vi "MeasureDistanceGantryCalibCheck.vi"() -> ()   [LabVIEW 2019]
uses:
  <vilib>/userDefined/High Color/IMAQdx.ctl
  include/GlobalVariables.vi
  Other Models/2010/Motion/AbortSingle.vi
  <vilib>/vision/driver/NI_Vision_Acquisition_Software.lvlib
panel:
  in  "TemplateFileName":string="C:\\Users\\TTUHEP\\Pictures\\SiCorner.png"
  out "X2Y2":string
  out "X1Y1":string
  in  "ObjectDetType":enum16{"Pattern", "ManualPick", "FidCircle"}(ring)
  in  "Gcode2":string="G90\nG1 Z0 F100\nG1 X224.526 Y907.397 F100//Si corner on BP A1\nG1 Z68.674 F100//Si Corner on BP A1\n//G1 X194.1280 Y755.823 F100 //Si Corner on BP A2\r//G1 Z68.8520934 //Si Corner on BP A1"
  in  "EnablePoint1":bool
  in  "Gcode1":string="G90\nG1 Z0 F100\nG1 X850.587 Y914.513 F100//Si corner A1\nG1 Z75.21 F100//Si Corner A1\n//G1 X768.633 Y750.333 F100 //Si corner A2\r//G1 Z75.0621//Si corner A2"
  in  "Operation2":enum16{"JoyStick", "FixedXY"}(ring)
  in  "Operation1":enum16{"JoyStick", "FixedXY"}(ring)
  out "CamX1Y1X2Y2Dist":string
  out "DistanceCam":dbl
  out "CamY 2":dbl
  out "CamX 2":dbl
  out "CamY":dbl
  out "CamX":dbl
  in  "EnablePoint2":bool
  out "error out":errorcluster
  out "X1Y1X2Y2Dist":string
  out "Distance":dbl
  out "Y2":dbl format="%#_7g"
  out "X2":dbl
  out "Radius 2":dbl
  out "CenterPosition 2":cluster{"X":sgl, "Y":sgl}
  in  "StopJoyStick 2":bool
  out "Image 2":T1(plugin-control)
  out "Y1":dbl format="%#_7g"
  out "X1":dbl
  out "Radius":dbl
  out "CenterPosition":cluster{"X":sgl, "Y":sgl}
  in  "StopJoyStick":bool
  in  "Autofocus":T2={"Enable"=TRUE, "InitialStepSize"=0.05, "Tolerance"=0.02, "Abort"=FALSE} {"Tolerance" format="%#_13g"}
  out "Image":T1(plugin-control)
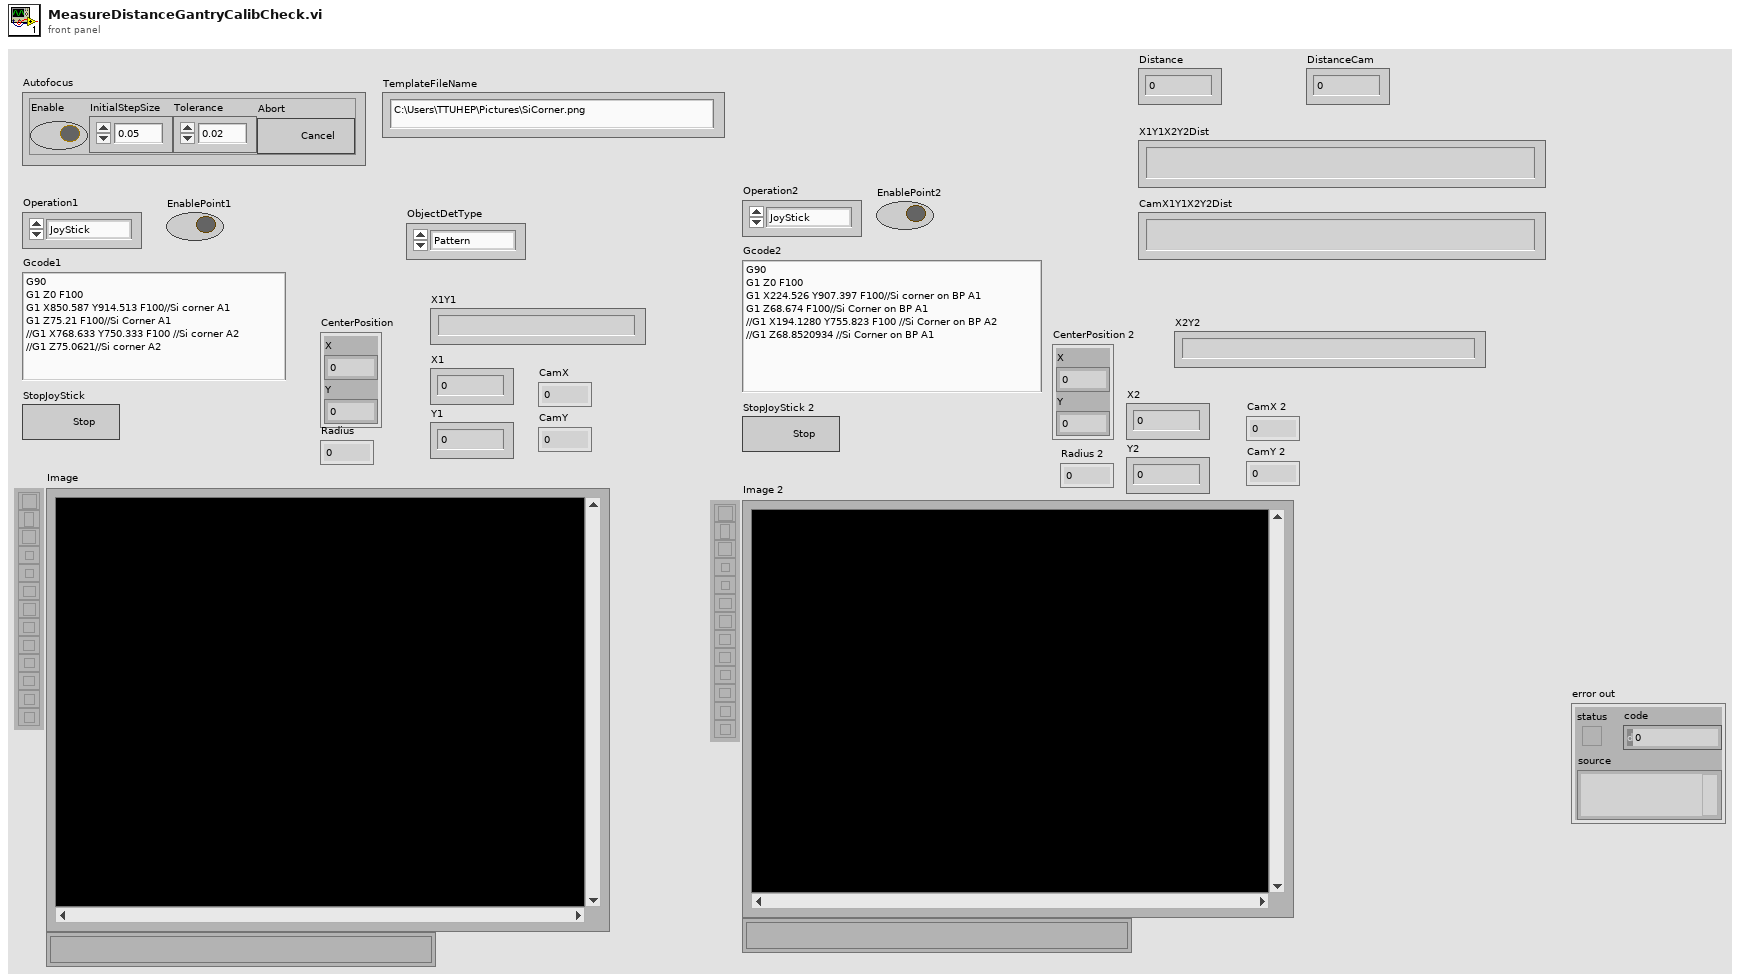
[diagram p1: front panel]
types:
  T1 = typedef "IMAQ Image.ctl" = refnum<image>
  T2 = cluster{"Enable":bool, "InitialStepSize":dbl, "Tolerance":dbl, "Abort":bool}
  T3 = typedef "IMAQdx.ctl" = refnum<k21>
  T4 = typedef "Image Type" = u32
  T5 = typedef "IMAQ Point" = cluster{"X":sgl, "Y":sgl}
  T6 = cluster{"Position":cluster{"X":sgl, "Y":sgl}, "Radius":dbl, "Score":dbl}
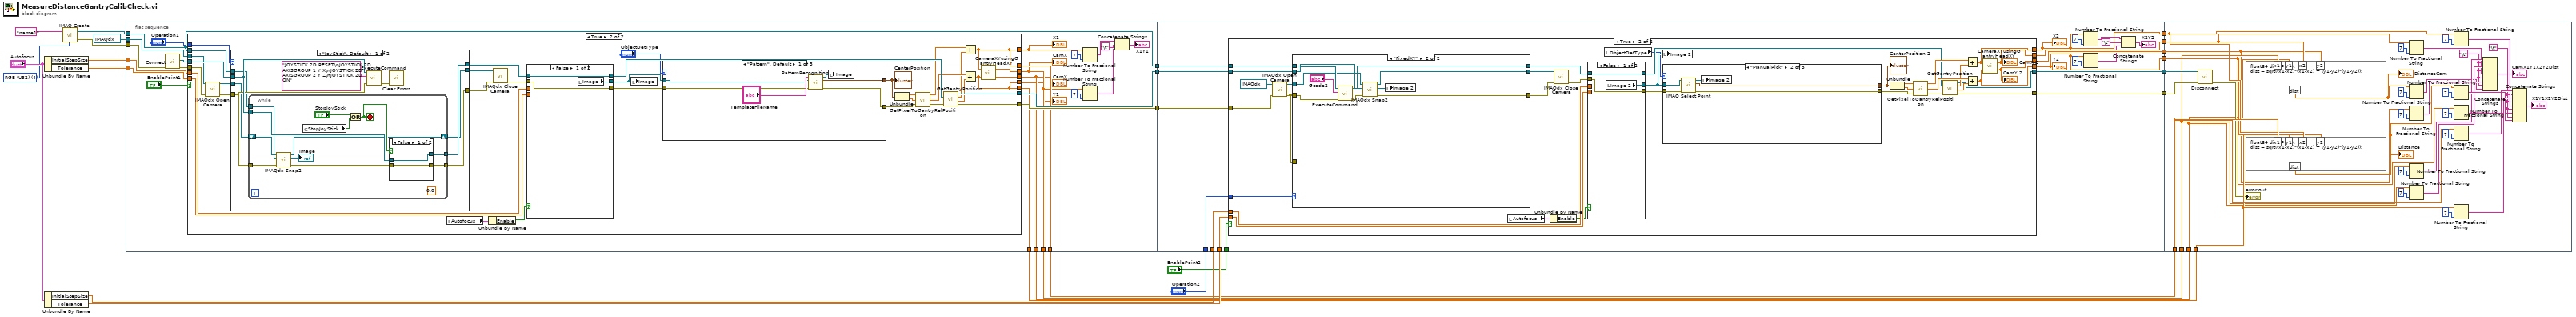
[diagram p0: block diagram]
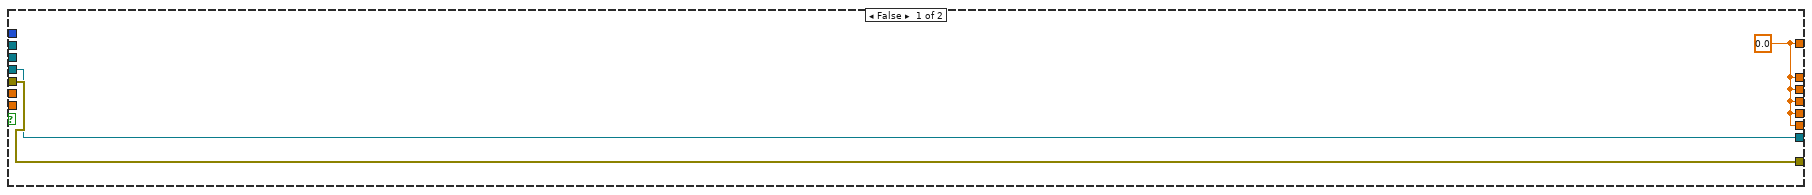
[diagram p2: hidden frame]
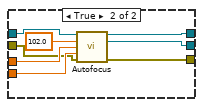
[diagram p3: hidden frame]
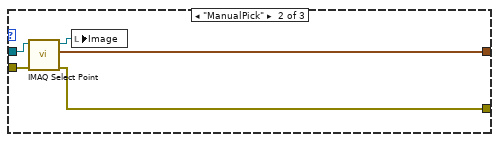
[diagram p4: hidden frame]
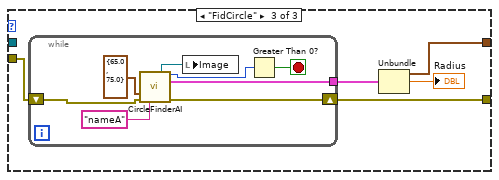
[diagram p5: hidden frame]
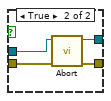
[diagram p6: hidden frame]
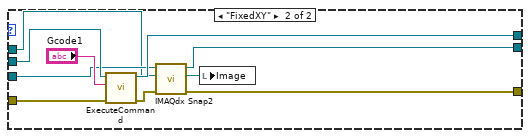
[diagram p7: hidden frame]
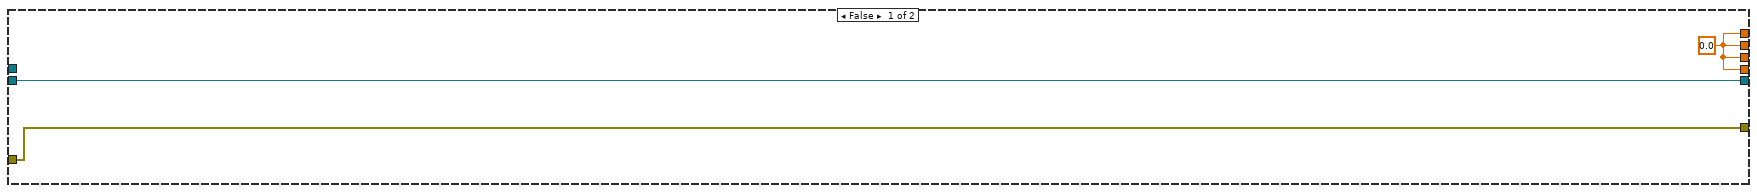
[diagram p8: hidden frame]
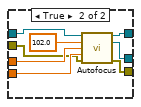
[diagram p9: hidden frame]
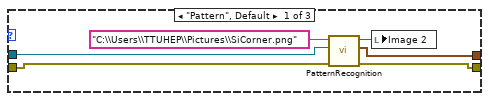
[diagram p10: hidden frame]
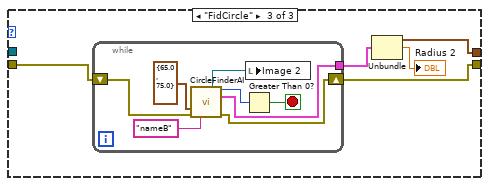
[diagram p11: hidden frame]
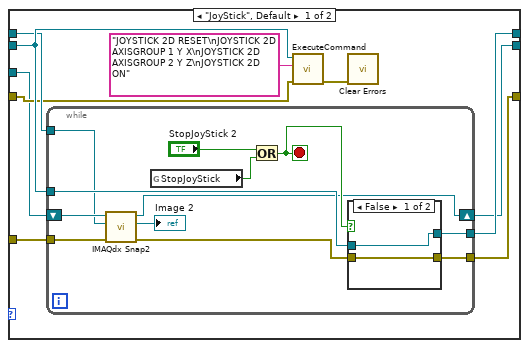
[diagram p12: hidden frame]
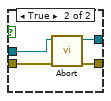
[diagram p13: hidden frame]
diagram:
  w13 = T4 4 items=["Grayscale (U8)", "Grayscale (I16)", "Grayscale (SGL)", "Complex (CSG)", "RGB (U32)", "HSL (U32)", "RGB (U64)", "Grayscale (U16)"] ("Image Type")
  n1 = Unbundle By Name("Autofocus") -> ("InitialStepSize"=w24:dbl, "Tolerance"=w25:dbl)
  n2 = Unbundle By Name("Autofocus") -> ("InitialStepSize"=w20:dbl, "Tolerance"=w19:dbl)
  n3 = call "IMAQ Create"("Image Name"="name1" ("ImageName"), "Image Type"=w13) -> ("New Image"=w12:T1, "error out"=w10:errorcluster)  [unwired: 3 in]
  n4 = flat-sequence {
    tunnel: w25 -> [w48]
    tunnel: w24 -> [w47]
    tunnel: [w44] -> w22
    tunnel: [w43] -> w21
    tunnel: [w41] -> w16
    tunnel: [w40] -> w15
    tunnel: w12 -> [w42]
    tunnel: [w42] -> w11
    tunnel: w10 -> [w34]
    tunnel: T3 "cam1" ("Camera") -> [w35]
    tunnel: [w39] -> w3
    tunnel: [w38] -> w2
    tunnel: w22 -> [w176]
    tunnel: w21 -> [w172]
    tunnel: w20 -> [w175]
    tunnel: w19 -> [w174]
    tunnel: [w159] -> w18
    tunnel: [w158] -> w17
    tunnel: w11 -> [w173]
    tunnel: [w171] -> w8
    tunnel: [w170] -> w7
    tunnel: "EnablePoint2" -> [w169]
    tunnel: [w168] -> w5
    tunnel: [w167] -> w4
    tunnel: "Operation2" -> [w166]
    tunnel: w18 -> [w314]
    tunnel: w17 -> [w313]
    tunnel: w16 -> [w320]
    tunnel: w15 -> [w315]
    tunnel: w8 -> [w323]
    tunnel: w7 -> [w322]
    tunnel: w5 -> [w289]
    tunnel: w4 -> [w288]
    tunnel: w3 -> [w291]
    tunnel: w2 -> [w290]
    frame #0 {
      n5 = call "Connect.vi"("error in (no error)"=w34) -> ("error out"=w45:errorcluster, "controller"=w46:refnum<k24>)  [unwired: 9 in]
      n6 = case shown="True" "EnablePoint1" {
        tunnel: w48 -> [_ w85]
        tunnel: w47 -> [_ w84]
        tunnel: w46 -> [w50 w83]
        tunnel: w45 -> [w51 w57]
        tunnel: [w50 w74] -> w44
        tunnel: [w51 w73] -> w43
        tunnel: w42 -> [_ w68]
        tunnel: [w49 w61] -> w41
        tunnel: [w49 w60] -> w40
        tunnel: [w49 w67] -> w39
        tunnel: [w49 w66] -> w38
        tunnel: "Operation1" -> [_ w65]
        tunnel: [w49 w61] -> w32
        tunnel: [w49 w60] -> w30
        tunnel: w35 -> [_ w59]
        frame False {
          w49 = 0.0
        }
        frame True {
          n7 = call <vilib>:"IMAQdx Open Camera.vi"("error in"=w57, "Session In"=w59) -> ("error out"=w56:errorcluster, "Session Out"=w58:T3)  [unwired: 8 in]
          n8 = case shown="\"JoyStick\", Default" w65 {
            tunnel: w83 -> [w128 w157]
            tunnel: [w126 w155] -> w82
            tunnel: w56 -> [w125 w156]
            tunnel: w68 -> [w124 w149]
            tunnel: w58 -> [w123 w153]
            tunnel: [w122 w151] -> w64
            tunnel: [w121 w150] -> w63
            frame "JoyStick", Default {
              n9 = while {
                tunnel: w128 -> [w141]
                tunnel: [w140] -> w122
                tunnel: [w139] -> w126
                tunnel: w125 -> [w135]
                shift-right: [w133] -> w121
                shift-left: w123 -> [w132]
                tunnel: w124 -> [w130]
                stop <- w136 stop-if-true
                (unwired) sgl 0.0 ("Rotate (degrees)")
                n10 = call <vilib>:"IMAQdx Snap2.vi"("error in"=w135, "Image In"=w130, "Session In"=w132) -> ("error out"=w131:errorcluster, "Image Out"=→"Image":T1, "Session Out"=w133:T3)  [unwired: 6 in]
                n11 = global read "GlobalVariables.vi" "StopJoyStick"() -> (w137:bool)
                n12 = Or(x="StopJoyStick", y=w137) -> (x .or. y?=w136:bool)
                n13 = case shown="False" w136 {
                  tunnel: w141 -> [w143 w147]
                  tunnel: w131 -> [w142 w146]
                  tunnel: [w142 w145] -> w140
                  tunnel: [w143 w144] -> w139
                  frame False {
                  }
                  frame True {
                    n14 = call-poly "Abort.vi"("error in (no error)"=w146, "controller in"=w147) -> ("error out"=w145:errorcluster, "controller out"=w144:refnum<k24>)  [unwired: 8 in]
                  }
                }
              }
              n15 = call "ExecuteCommand.vi"("error in (no error)"=w125, "Command Code"="JOYSTICK 2D RESET\nJOYSTICK 2D AXISGROUP 1 Y X\nJOYSTICK 2D AXISGROUP 2 Y Z\nJOYSTICK 2D ON", "controller in"=w128) -> ("error out"=w127:errorcluster)  [unwired: 6 in, 2 out]
              n16 = call <vilib>:"Clear Errors.vi"("error in (no error)"=w127) -> ()  [unwired: 5 in, 2 out]
            }
            frame "FixedXY" {
              n17 = call "ExecuteCommand.vi"("error in (no error)"=w156, "Command Code"="Gcode1", "controller in"=w157) -> ("error out"=w152:errorcluster, "controller out"=w155:refnum<k24>)  [unwired: 6 in, 1 out]
              n18 = call <vilib>:"IMAQdx Snap2.vi"("error in"=w152, "Image In"=w149, "Session In"=w153) -> ("error out"=w151:errorcluster, "Image Out"=w148:T1, "Session Out"=w150:T3)  [unwired: 6 in]
              n19 = local write "Image"(w148) -> ()
            }
          }
          n20 = local read "Autofocus"() -> (w53:T2)
          n21 = Unbundle By Name(w53) -> ("Enable"=w52:bool)
          n22 = call <vilib>:"IMAQdx Close Camera.vi"("error in"=w64, "Session In"=w63) -> ("error out"=w62:errorcluster)  [unwired: 9 in]
          n23 = case shown="False" w52 {
            tunnel: w85 -> [_ w95]
            tunnel: w84 -> [_ w94]
            tunnel: w82 -> [w87 w93]
            tunnel: [w88 w92] -> w81
            tunnel: [w87 w91] -> w80
            tunnel: w62 -> [w88 w90]
            tunnel: [w86 w89] -> w55
            frame False {
              n24 = local read "Image"() -> (w86:T1)
            }
            frame True {
              n25 = call "Autofocus.vi"("controller in"=w93, "SafeMaxZ"=102.0, "InitialStepSize"=w94, "Tolerance"=w95, "error in (no error)"=w90) -> ("controller out"=w91:refnum<k24>, "Image"=w89:T1, "error out"=w92:errorcluster)  [unwired: 5 in, 3 out]
            }
          }
          n26 = local write "Image"(w55) -> ()
          n27 = case shown="\"Pattern\", Default" "ObjectDetType" {
            tunnel: w81 -> [w97 w104 w112]
            tunnel: [w98 w106 w109] -> w79
            tunnel: [w99 w105 w108] -> w76
            tunnel: w55 -> [w101 w107 _]
            frame "Pattern", Default {
              n28 = call "PatternRecognition.vi"("error in (no error)"=w97, "ImageIn"=w101, "TemplateFileName"="TemplateFileName") -> ("error out"=w99:errorcluster, "Position"=w98:cluster{"x":sgl, "y":sgl}, "ImageFoundPattern"=w100:T1)  [unwired: 3 in, 2 out]
              n29 = local write "Image"(w100) -> ()
            }
            frame "ManualPick" {
              n30 = call "IMAQ Select Point"("error in (no error)"=w104, "Image In"=w107) -> ("error out"=w105:errorcluster, "Point"=w106:T5, "Image Out (duplicate)"=w103:T1)  [unwired: 6 in, 1 out]
              n31 = local write "Image"(w103) -> ()
            }
            frame "FidCircle" {
              n32 = while {
                tunnel: [w117] -> w111
                shift-right: [w116] -> w108
                shift-left: w112 -> [w118]
                stop <- w113 stop-if-true
                n33 = call "CircleFinderAI.vi"("Circle Descriptor"=cluster{"Min Radius":dbl, "Max Radius":dbl} {"Min Radius"=65.0, "Max Radius"=75.0}, "error in (no error)"=w118, "Image Name"="nameA") -> ("Image"=w115:T1, "NumCirclesFound"=w114:i32, "Circle0"=w117:T6, "error out"=w116:errorcluster)  [unwired: 7 in, 2 out]
                n34 = local write "Image"(w115) -> ()
                n35 = Greater Than 0?(x=w114) -> (x > 0?=w113:bool)
              }
              n36 = Unbundle(w111) -> ("Position"=w109:cluster{"X":sgl, "Y":sgl}, "Radius"=→"Radius":dbl)  [unwired: 1 out]
            }
          }
          "CenterPosition" <- w79
          n37 = Unbundle(w79) -> ("X"=w78:sgl, "Y"=w77:sgl)
          n38 = call "GetPixelToGantryRelPosition.vi"("error in (no error)"=w76, "PixelY"=w77, "PixelX"=w78) -> ("error out"=w75:errorcluster, "YmmRelGH"=w71:dbl, "XmmRelGH"=w69:dbl)
          n39 = call "GetGantryPosition.vi"("error in (no error)"=w75, "Controller In"=w80) -> ("error out"=w73:errorcluster, "Position Y"=w72:dbl, "Position X"=w70:dbl, "controller out"=w74:refnum<k24>)  [unwired: 3 in, 3 out]
          n40 = Add(x=w69, y=w70) -> (x+y=w61:dbl)
          n41 = Add(x=w71, y=w72) -> (x+y=w60:dbl)
          n42 = call "CameraXYusingGantryHeadXY.vi"("GantryY"=w60, "GantryX"=w61) -> ("CamY"=w66:dbl, "CamX"=w67:dbl)
        }
      }
      "CamX" <- w39
      "CamY" <- w38
      "X1" <- w32
      "Y1" <- w30
      n43 = Number To Fractional String(number=w32, precision (6)=i16 7) -> (F-format string=w29:string)  [unwired: 2 in]
      n44 = Number To Fractional String(number=w30, precision (6)=i16 7) -> (F-format string=w27:string)  [unwired: 2 in]
      n45 = Concatenate Strings(w29, "\t", w27) -> (→"X1Y1":string)
    }
    frame #1 {
      n46 = case shown="True" w169 {
        tunnel: w176 -> [w178 w213]
        tunnel: w175 -> [_ w200]
        tunnel: w174 -> [_ w199]
        tunnel: [w177 w192] -> w159
        tunnel: [w177 w191] -> w158
        tunnel: w173 -> [_ w195]
        tunnel: w172 -> [w179 w187]
        tunnel: [w178 w194] -> w171
        tunnel: [w179 w193] -> w170
        tunnel: [w177 w190] -> w168
        tunnel: [w177 w189] -> w167
        tunnel: w166 -> [_ w188]
        frame False {
          w177 = 0.0
        }
        frame True {
          n47 = call <vilib>:"IMAQdx Open Camera.vi"("error in"=w187, "Session In"=T3 "cam1") -> ("error out"=w185:errorcluster, "Session Out"=w184:T3)  [unwired: 8 in]
          n48 = case shown="\"FixedXY\"" w188 {
            tunnel: w213 -> [w258 w285]
            tunnel: [w255 w284] -> w201
            tunnel: [w254 w278] -> w198
            tunnel: [w253 w279] -> w197
            tunnel: w195 -> [w252 w282]
            tunnel: w185 -> [w251 w280]
            tunnel: w185 -> [w250 _]
            tunnel: w184 -> [w249 w283]
            frame "JoyStick", Default {
              n49 = while {
                tunnel: w258 -> [w270]
                tunnel: [w269] -> w253
                tunnel: [w268] -> w255
                shift-right: [w263] -> w254
                shift-left: w249 -> [w264]
                tunnel: w252 -> [w260]
                tunnel: w250 -> [w259]
                stop <- w265 stop-if-true
                n50 = call <vilib>:"IMAQdx Snap2.vi"("error in"=w259, "Image In"=w260, "Session In"=w264) -> ("error out"=w261:errorcluster, "Image Out"=→"Image 2":T1, "Session Out"=w263:T3)  [unwired: 6 in]
                n51 = global read "GlobalVariables.vi" "StopJoyStick"() -> (w266:bool)
                n52 = Or(x="StopJoyStick 2", y=w266) -> (x .or. y?=w265:bool)
                n53 = case shown="False" w265 {
                  tunnel: w270 -> [w272 w276]
                  tunnel: w261 -> [w271 w275]
                  tunnel: [w271 w274] -> w269
                  tunnel: [w272 w273] -> w268
                  frame False {
                  }
                  frame True {
                    n54 = call-poly "Abort.vi"("error in (no error)"=w275, "controller in"=w276) -> ("error out"=w274:errorcluster, "controller out"=w273:refnum<k24>)  [unwired: 8 in]
                  }
                }
              }
              n55 = call "ExecuteCommand.vi"("error in (no error)"=w251, "Command Code"="JOYSTICK 2D RESET\nJOYSTICK 2D AXISGROUP 1 Y X\nJOYSTICK 2D AXISGROUP 2 Y Z\nJOYSTICK 2D ON", "controller in"=w258) -> ("error out"=w257:errorcluster)  [unwired: 6 in, 2 out]
              n56 = call <vilib>:"Clear Errors.vi"("error in (no error)"=w257) -> ()  [unwired: 5 in, 2 out]
            }
            frame "FixedXY" {
              n57 = call "ExecuteCommand.vi"("error in (no error)"=w280, "Command Code"="Gcode2", "controller in"=w285) -> ("error out"=w281:errorcluster, "controller out"=w284:refnum<k24>)  [unwired: 6 in, 1 out]
              n58 = call <vilib>:"IMAQdx Snap2.vi"("error in"=w281, "Image In"=w282, "Session In"=w283) -> ("error out"=w279:errorcluster, "Image Out"=w277:T1, "Session Out"=w278:T3)  [unwired: 6 in]
              n59 = local write "Image 2"(w277) -> ()
            }
          }
          n60 = local read "Autofocus"() -> (w181:T2)
          n61 = Unbundle By Name(w181) -> ("Enable"=w180:bool)
          n62 = call <vilib>:"IMAQdx Close Camera.vi"("error in"=w197, "Session In"=w198) -> ("error out"=w196:errorcluster)  [unwired: 9 in]
          n63 = case shown="False" w180 {
            tunnel: [w215 w224] -> w203
            tunnel: [w216 w223] -> w202
            tunnel: w201 -> [w215 w222]
            tunnel: w200 -> [_ w220]
            tunnel: w199 -> [_ w219]
            tunnel: w196 -> [w216 w218]
            tunnel: [w214 w217] -> w183
            frame False {
              n64 = local read "Image 2"() -> (w214:T1)
            }
            frame True {
              n65 = call "Autofocus.vi"("controller in"=w222, "SafeMaxZ"=102.0, "InitialStepSize"=w220, "Tolerance"=w219, "error in (no error)"=w218) -> ("controller out"=w224:refnum<k24>, "Image"=w217:T1, "error out"=w223:errorcluster)  [unwired: 5 in, 3 out]
            }
          }
          n66 = local read "ObjectDetType"() -> (w182:enum16{"Pattern", "ManualPick", "FidCircle"})
          n67 = local write "Image 2"(w183) -> ()
          n68 = case shown="\"ManualPick\"" w182 {
            tunnel: [w227 w233 w240] -> w207
            tunnel: [w225 w232 w239] -> w204
            tunnel: w202 -> [w228 w234 w236]
            tunnel: w183 -> [w229 w235 _]
            frame "Pattern", Default {
              n69 = call "PatternRecognition.vi"("error in (no error)"=w228, "ImageIn"=w229, "TemplateFileName"="C:\\Users\\TTUHEP\\Pictures\\SiCorner.png") -> ("error out"=w227:errorcluster, "Position"=w225:cluster{"x":sgl, "y":sgl}, "ImageFoundPattern"=w226:T1)  [unwired: 3 in, 2 out]
              n70 = local write "Image 2"(w226) -> ()
            }
            frame "ManualPick" {
              n71 = call "IMAQ Select Point"("error in (no error)"=w234, "Image In"=w235) -> ("error out"=w233:errorcluster, "Point"=w232:T5, "Image Out (duplicate)"=w231:T1)  [unwired: 6 in, 1 out]
              n72 = local write "Image 2"(w231) -> ()
            }
            frame "FidCircle" {
              n73 = while {
                tunnel: [w247] -> w237
                shift-right: [w248] -> w240
                shift-left: w236 -> [w246]
                stop <- w241 stop-if-true
                n74 = call "CircleFinderAI.vi"("Circle Descriptor"=cluster{"Min Radius":dbl, "Max Radius":dbl} {"Min Radius"=65.0, "Max Radius"=75.0}, "error in (no error)"=w246, "Image Name"="nameB") -> ("Image"=w244:T1, "NumCirclesFound"=w242:i32, "Circle0"=w247:T6, "error out"=w248:errorcluster)  [unwired: 7 in, 2 out]
                n75 = Greater Than 0?(x=w242) -> (x > 0?=w241:bool)
                n76 = local write "Image 2"(w244) -> ()
              }
              n77 = Unbundle(w237) -> ("Position"=w239:cluster{"X":sgl, "Y":sgl}, "Radius"=→"Radius 2":dbl)  [unwired: 1 out]
            }
          }
          "CenterPosition 2" <- w204
          n78 = Unbundle(w204) -> ("X"=w205:sgl, "Y"=w206:sgl)
          n79 = call "GetPixelToGantryRelPosition.vi"("error in (no error)"=w207, "PixelY"=w206, "PixelX"=w205) -> ("error out"=w208:errorcluster, "YmmRelGH"=w211:dbl, "XmmRelGH"=w209:dbl)
          n80 = call "GetGantryPosition.vi"("error in (no error)"=w208, "Controller In"=w203) -> ("error out"=w193:errorcluster, "Position Y"=w212:dbl, "Position X"=w210:dbl, "controller out"=w194:refnum<k24>)  [unwired: 3 in, 3 out]
          n81 = Add(x=w209, y=w210) -> (x+y=w192:dbl)
          n82 = Add(x=w211, y=w212) -> (x+y=w191:dbl)
          n83 = call "CameraXYusingGantryHeadXY.vi"("GantryY"=w191, "GantryX"=w192) -> ("CamY"=w189:dbl, "CamX"=w190:dbl)
          "CamX 2" <- w190
          "CamY 2" <- w189
        }
      }
      "X2" <- w159
      "Y2" <- w158
      n84 = Number To Fractional String(number=w159, precision (6)=i16 7) -> (F-format string=w163:string)  [unwired: 2 in]
      n85 = Number To Fractional String(number=w158, precision (6)=i16 7) -> (F-format string=w161:string)  [unwired: 2 in]
      n86 = Concatenate Strings(w163, "\t", w161) -> (→"X2Y2":string)
    }
    frame #2 {
      w294 = "\t"
      w307 = "\t"
      n87 = call "Disconnect.vi"("error in (no error)"=w322, "controller"=w323) -> ("error out"=→"error out":errorcluster)  [unwired: 9 in]
      n88 = formula code="float64 dist = 0.0;\ndist = sqrt((x1-x2)*(x1-x2) + (y1-y2)*(y1-y2));"("x1"=w291, "y1"=w290, "x2"=w289, "y2"=w288) -> ("dist"=w287:dbl)
      "DistanceCam" <- w287
      n89 = formula code="float64 dist = 0.0;\ndist = sqrt((x1-x2)*(x1-x2) + (y1-y2)*(y1-y2));"("x1"=w320, "y1"=w315, "x2"=w314, "y2"=w313) -> ("dist"=w312:dbl)
      "Distance" <- w312
      n90 = Number To Fractional String(number=w289, precision (6)=i16 7) -> (F-format string=w296:string)  [unwired: 2 in]
      n91 = Number To Fractional String(number=w287, precision (6)=i16 7) -> (F-format string=w293:string)  [unwired: 2 in]
      n92 = Number To Fractional String(number=w288, precision (6)=i16 7) -> (F-format string=w295:string)  [unwired: 2 in]
      n93 = Number To Fractional String(number=w291, precision (6)=i16 7) -> (F-format string=w298:string)  [unwired: 2 in]
      n94 = Number To Fractional String(number=w290, precision (6)=i16 7) -> (F-format string=w297:string)  [unwired: 2 in]
      n95 = Number To Fractional String(number=w314, precision (6)=i16 7) -> (F-format string=w309:string)  [unwired: 2 in]
      n96 = Number To Fractional String(number=w312, precision (6)=i16 7) -> (F-format string=w306:string)  [unwired: 2 in]
      n97 = Number To Fractional String(number=w313, precision (6)=i16 7) -> (F-format string=w308:string)  [unwired: 2 in]
      n98 = Number To Fractional String(number=w320, precision (6)=i16 7) -> (F-format string=w311:string)  [unwired: 2 in]
      n99 = Number To Fractional String(number=w315, precision (6)=i16 7) -> (F-format string=w310:string)  [unwired: 2 in]
      n100 = Concatenate Strings(w298, w294, w297, w294, w296, w294, w295, w294, w293) -> (→"CamX1Y1X2Y2Dist":string)
      n101 = Concatenate Strings(w311, w307, w310, w307, w309, w307, w308, w307, w306) -> (→"X1Y1X2Y2Dist":string)
    }
  }
